vi "Read Magnetic Deviation.vi"(8 "error in (no error)":errorcluster, 11 "Compass Instrument in":refnum<class "Compass Instrument.lvclass">) -> (0 "error out":errorcluster, 2 "Magnetic Deviation":dbl, 3 "Compass Instrument out":refnum<class "Compass Instrument.lvclass">)   [LabVIEW 2015, in "Compass Instrument.lvlib" / "Compass Instrument.lvclass"]
uses:
  Compass Instrument.lvclass
  Compass Instrument.lvclass/Compass Instrument.ctl
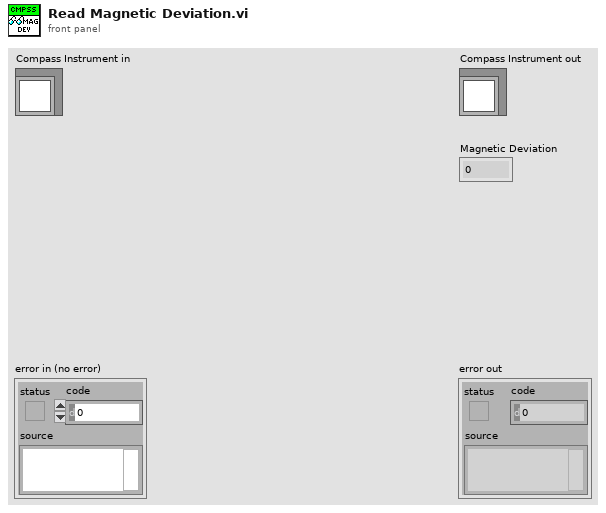
[diagram p1: front panel]
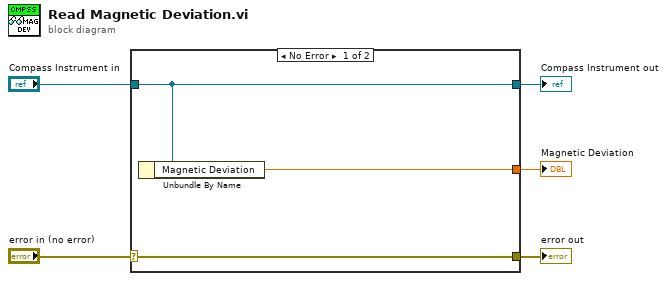
[diagram p0: block diagram]
diagram:
  n1 = case shown="No Error" "error in (no error)" {
    selector: "error in (no error)" -> [w8 w9]
    tunnel: [w8 w9] -> w4
    tunnel: [w7 w10] -> w2
    tunnel: "Compass Instrument in" -> [w7 w10]
    tunnel: [w6 _] -> w1
    frame No Error {
      n2 = Unbundle By Name(w7) -> ("Magnetic Deviation"=w6:sgl)
    }
    frame Error {
    }
  }
  "error out" <- w4
  "Compass Instrument out" <- w2
  "Magnetic Deviation" <- w1
